vi "DefaultPanel.vi"() -> ()   [LabVIEW 2020]
panel:
  in  "stop":bool
  # "Welcome to ARCOS\nWait For Insert User Panel"
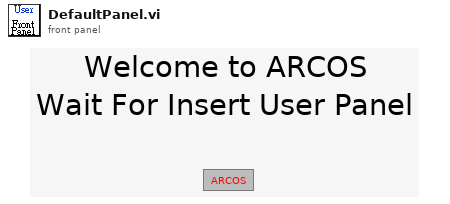
[diagram p1: front panel]
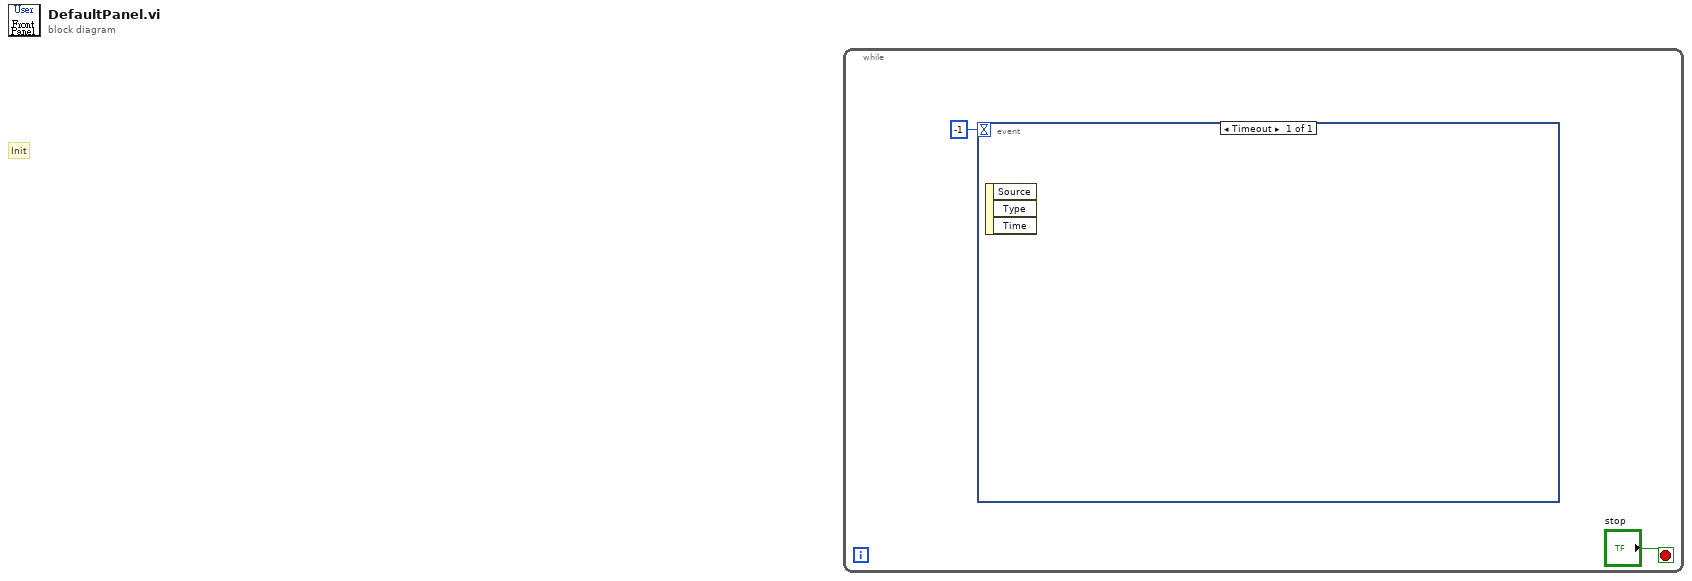
[diagram p0: block diagram]
diagram:
  # "Init"
  n1 = while {
    stop <- "stop" stop-if-true
    n2 = event shown="[0] Timeout" {
      selector: _ -> [_]
      dyn-events: _ -> [_]
      timeout: -1 -> [_]
      event Timeout {
        n3 = event-data() -> ()  [unwired: 1 in, 3 out]
      }
    }
  }
